vi "Get GPS Data.vi"(8 "error in":errorcluster, 11 "FPGA_MAIN ref in":T1) -> (0 "error out":errorcluster, 2 "GPS Point":T2 {"Longitude" format="%#_14g"; "Latitude" format="%#_14g"}, 3 "FPGA_MAIN ref out":T1)   [LabVIEW 2009]
uses:
  TypeDefs/Sensor TypeDefs/GPS Data.ctl
  TypeDefs/Sensor TypeDefs/FPGA Main ref.ctl
  <vilib>/rvi/interface/nirviReadWriteControl/nirviReadWriteControl.xnode
  FPGA Bitfiles/Q_IGVC_2010.lvproj_FPGA Target_FPGA_MAIN.vi.lvbitx
  <vilib>/LabVIEW Targets/FPGA/RIO/nirio_HostInterface/nirio_ReadBig.vi
  <vilib>/Utility/error.llb/Error Cluster From Error Code.vi
  <vilib>/rvi/errors/niLvFpgaAdjustHostInterfaceError.vi
  <vilib>/rvi/interface/common/niFpgaNodeNameForErrorReporting.ctl
  <vilib>/rvi/errors/niLvFpgaWhatHappensToTopLevelVI.ctl
  NiRioSrv.dll
panel:
  out "GPS error out":errorcluster
  out "New GPS Data":bool
  out "Bytes at Port?":bool
  out "Time":dbl format="%#_14g"
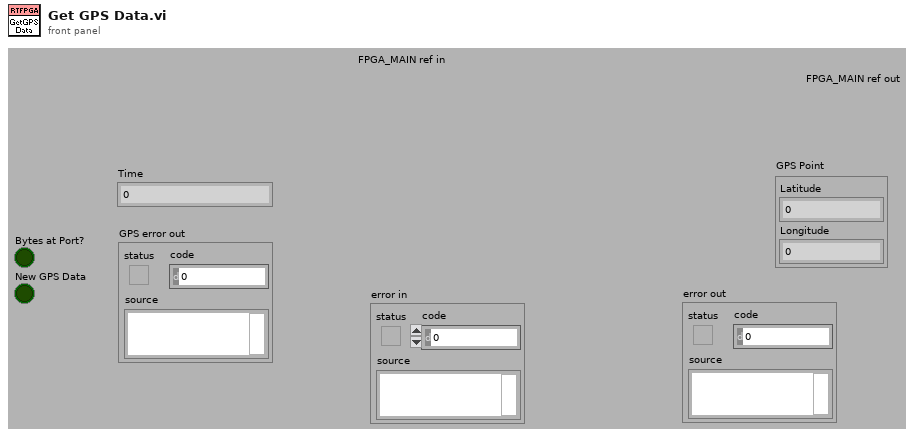
[diagram p1: front panel]
types:
  T1 = typedef "FPGA Main ref.ctl" = refnum<k20>
  T2 = typedef "GPS Data.ctl" = cluster{"Latitude":dbl, "Longitude":dbl}
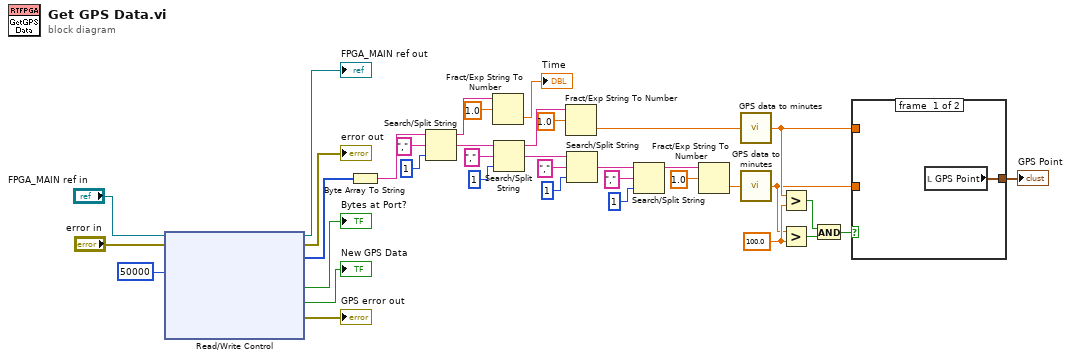
[diagram p0: block diagram]
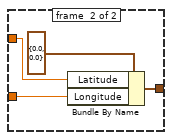
[diagram p2: hidden frame]
diagram:
  w7 = 100.0 ("y")
  n1 = xnode "Read/Write Control"("FPGA VI Reference In"="FPGA_MAIN ref in", "error in"="error in", "GPS Read Timeout (us)"=50000) -> ("FPGA VI Reference Out"=→"FPGA_MAIN ref out":T1, "error out"=→"error out":errorcluster, "GPS Data"=w20:u8[], "Bytes at Port?"=→"Bytes at Port?":bool, "New GPS Data"=→"New GPS Data":bool, "GPS error out"=→"GPS error out":errorcluster)  [unwired: 1 out]
  n2 = Byte Array To String(unsigned byte array=w20) -> (string=w15:string)
  n3 = Search/Split String(string=w15, search string/char (-)=",", offset (0)=1) -> (substring before match=w24:string, match + rest of string=w31:string)  [unwired: 1 out]
  n4 = Fract/Exp String To Number(string=w24, offset=1.0 ("default (0 I32)")) -> (number=→"Time":dbl)  [unwired: 2 in, 1 out]
  n5 = Search/Split String(string=w31, search string/char (-)=",", offset (0)=1) -> (substring before match=w26:string, match + rest of string=w30:string)  [unwired: 1 out]
  n6 = Fract/Exp String To Number(string=w26, offset=1.0 ("default (0 DBL)")) -> (number=w9:dbl)  [unwired: 2 in, 1 out]
  n7 = Search/Split String(string=w30, search string/char (-)=",", offset (0)=1) -> (match + rest of string=w27:string)  [unwired: 2 out]
  n8 = Search/Split String(string=w27, search string/char (-)=",", offset (0)=1) -> (substring before match=w19:string)  [unwired: 2 out]
  n9 = Fract/Exp String To Number(string=w19, offset=1.0 ("default (0 I32)")) -> (number=w8:dbl)  [unwired: 2 in, 1 out]
  n10 = call "GPS data to minutes.vi"("GPS Data in (DDmm.mm)"=w9) -> ("GPS Data out (in minutes)"=w3:dbl)
  n11 = call "GPS data to minutes.vi"("GPS Data in (DDmm.mm)"=w8) -> ("GPS Data out (in minutes)"=w2:dbl)
  n12 = Greater?(x=w3, y=w7) -> (0:w6:bool)
  n13 = Greater?(x=w2, y=w7) -> (0:w5:bool)
  n14 = And(x=w6, y=w5) -> (x .and. y?=w4:bool)
  n15 = case shown="False" w4 {
    tunnel: w3 -> [_ w41]
    tunnel: w2 -> [_ w40]
    tunnel: [w38 w39] -> w1
    frame #0 {
      n16 = local read "GPS Point"() -> (w38:T2)
    }
    frame #1 {
      n17 = Bundle By Name(cluster=T2 {"Latitude"=0.0, "Longitude"=0.0} ("GPS Point"), "Latitude"=w41, "Longitude"=w40) -> (w39:T2)
    }
  }
  "GPS Point" <- w1
